vi "MGCC_MdlMgmt_Vpu_slack_phase.vi"() -> ()   [LabVIEW 2016]
doc: "This VI is designed to initize the SHE215 model with Vpu slack phase (1D complex array)."
uses:
  <vilib>/imath/engines/lvmath2/RunTimeEngine/NodeEndStatement/NIMS_NodeEndStatement_Output.vi
  <instcachedir>/0/NIMS_NodeEndStatement_Output_53EC0D466D134D7ABD903AC30B43404B.lvgen/NIMS_NodeEndStatement_Output_53EC0D466D134D7ABD903AC30B43404B_000.vi
  <vilib>/imath/engines/lvmath2/RunTimeEngine/ErrorHandling/NIMS_Finalize Error.vi
  <vilib>/Utility/file.llb/Read Delimited Spreadsheet (string).vi
panel:
  out "all rows":string[][](array[string])
  out "Array":cdb[](array[numeric])
  out "text":string
  out "Vpu_slack_phase":cdb[](array[numeric])
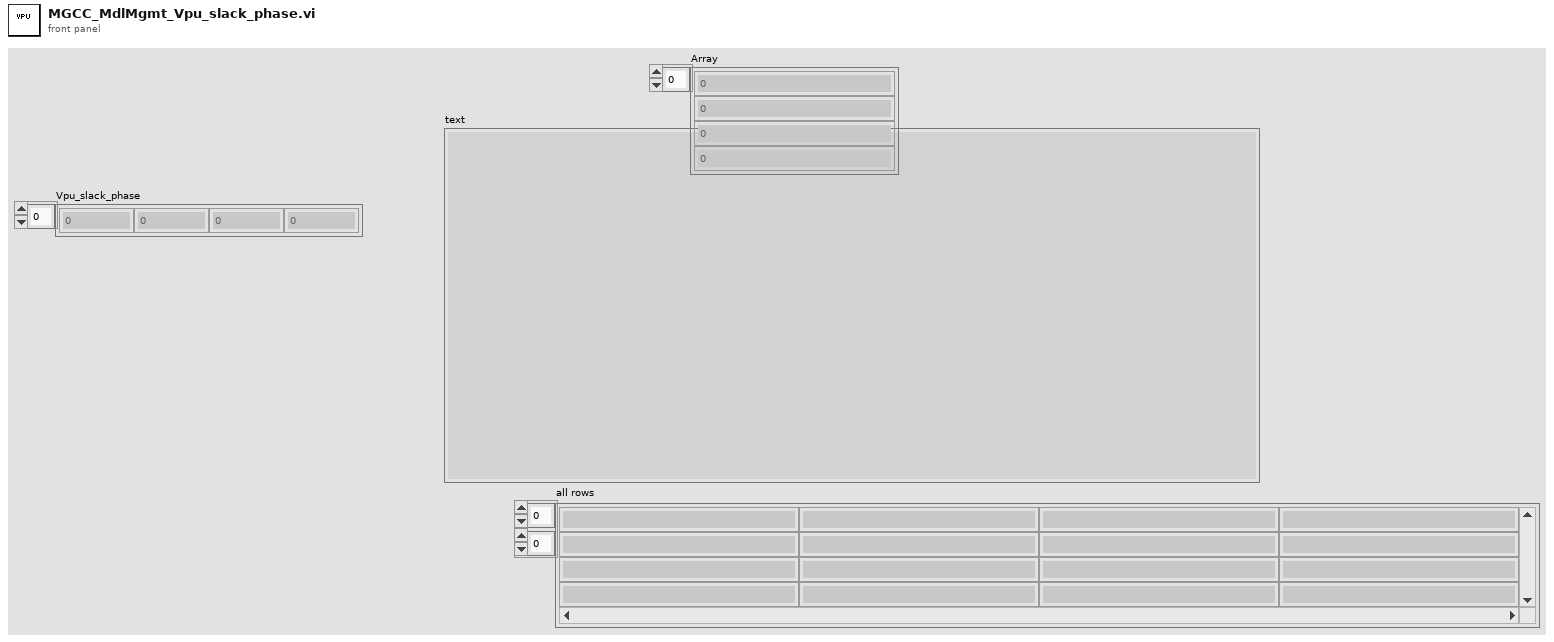
[diagram p1: front panel]
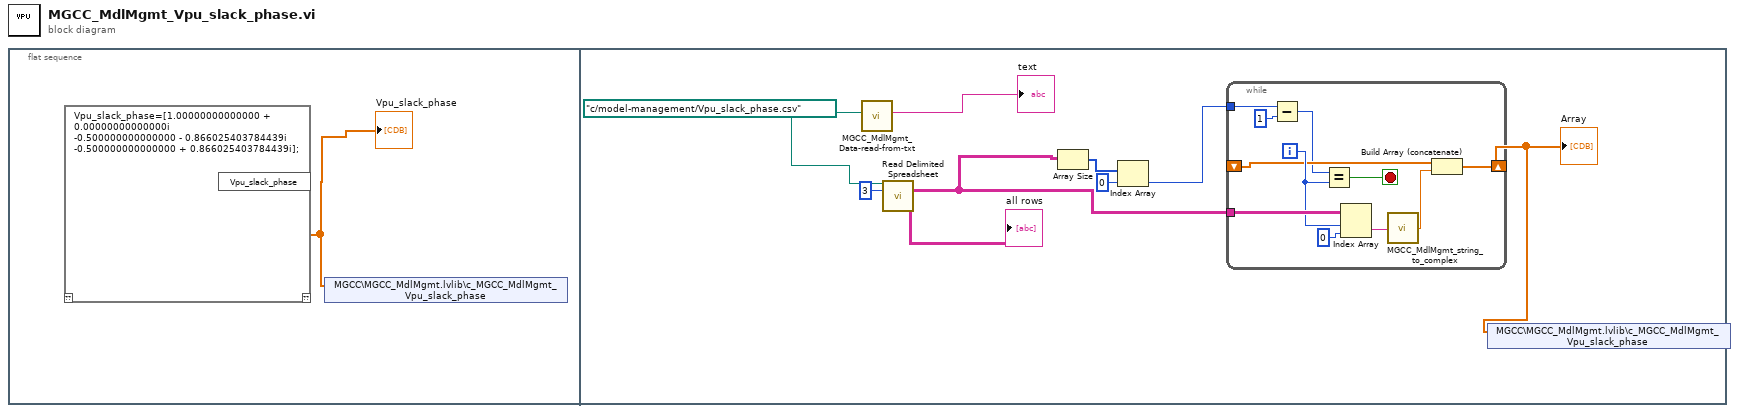
[diagram p0: block diagram]
diagram:
  n1 = flat-sequence {
    frame #0 {
      n2 = mathscript code="Vpu_slack_phase=[1.00000000000000 + 0.00000000000000i\n-0.500000000000000 - 0.866025403784439i\n-0.500000000000000 + 0.866025403784439i];"() -> ("Vpu_slack_phase"=w1:cdb[])  [unwired: 1 in, 1 out]
      "Vpu_slack_phase" <- w1
      n3 = shared-variable "MGCC\\MGCC_MdlMgmt.lvlib\\c_MGCC_MdlMgmt_Vpu_slack_phase"(w1) -> ()  [unwired: 1 in, 1 out]
    }
    frame #1 {
      w31 = path "c:/model-management/Vpu_slack_phase.csv" ("file path (use dialog)")
      n4 = call "MGCC_MdlMgmt_Data-read-from-txt.vi"("file path (use dialog)"=w31) -> ("text"=→"text":string)  [unwired: 10 in]
      n5 = call-poly <vilib>:"Read Delimited Spreadsheet.vi"("file path (dialog if empty)"=w31, "number of rows (all:-1)"=3) -> ("all rows"=w26:string[][])  [unwired: 8 in, 5 out]
      "all rows" <- w26
      n6 = Array Size(array=w26) -> (size(s)=w28:i32[])
      n7 = Index Array(array=w28, index=0) -> (element=w25:i32)
      n8 = while {
        tunnel: w26 -> [w40]
        tunnel: w25 -> [w35]
        shift-right: [w37] -> w24
        shift-left: _ -> [w36]
        i -> [w38]
        stop <- w42 stop-if-true
        n9 = Subtract(x=w35, y=1) -> (x-y=w33:i32)
        n10 = Equal?(x=w33, y=w38) -> (x = y?=w42:bool)
        n11 = Index Array(array=w40, index (row)=w38, index (col)=0 ("disabled index (col)")) -> (element=w32:string)
        n12 = call "MGCC_MdlMgmt_string_to_complex.vi"("String Input"=w32) -> ("Complex Number"=w41:cdb)
        n13 = Build Array (concatenate)(w36, w41) -> (w37:cdb[])
      }
      "Array" <- w24
      n14 = shared-variable "MGCC\\MGCC_MdlMgmt.lvlib\\c_MGCC_MdlMgmt_Vpu_slack_phase"(w24) -> ()  [unwired: 1 in, 1 out]
    }
  }
